vi "Escolher sinal.vi"(6 "Offset":dbl, 7 "Fase da onda":dbl, 9 "Numeric":dbl, 10 "Tipo de onda":T1, 11 "Amplitude":dbl) -> (3 "Sawtooth":dynamicdata(waveform))   [LabVIEW 2014]
uses:
  Tipos de onda.ctl
  <vilib>/measure/NI_MAPro.lvlib
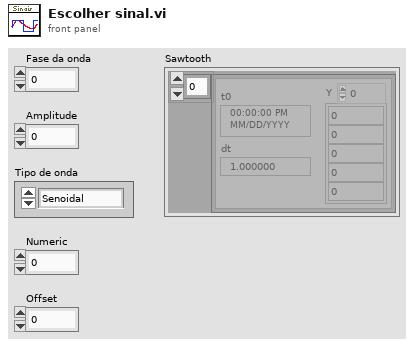
[diagram p1: front panel]
types:
  T1 = typedef "Tipos de onda.ctl" = enum16{"Senoidal", "Quadrada", "Triangular", "Trapezoidal", "Dente de Serra"}
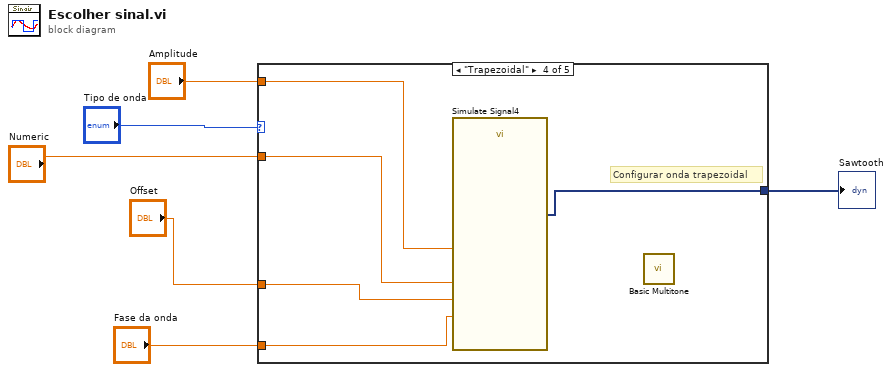
[diagram p0: block diagram]
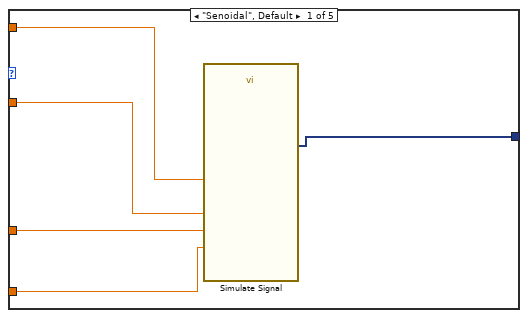
[diagram p2: hidden frame]
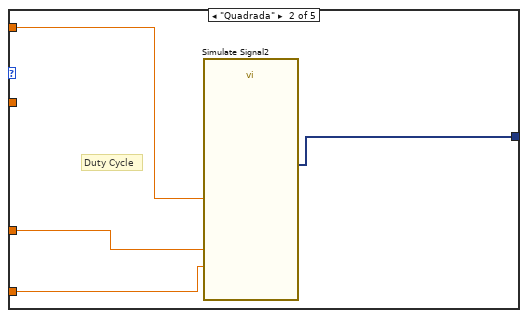
[diagram p3: hidden frame]
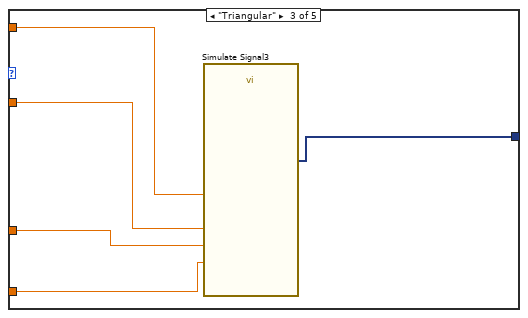
[diagram p4: hidden frame]
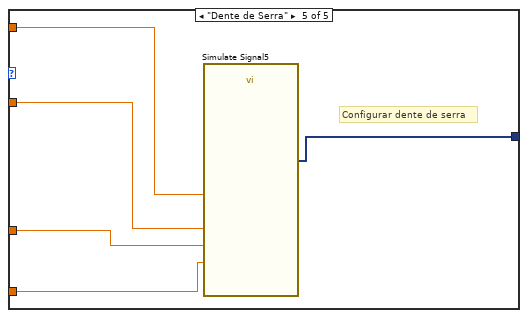
[diagram p5: hidden frame]
diagram:
  n1 = case shown="\"Trapezoidal\"" "Tipo de onda" {
    tunnel: "Amplitude" -> [w11 w15 w20 w25 w30]
    tunnel: "Numeric" -> [w10 _ w19 w24 w29]
    tunnel: "Fase da onda" -> [w9 w14 w18 w23 w28]
    tunnel: "Offset" -> [w8 w13 w17 w22 w27]
    tunnel: [w7 w12 w16 w21 w26] -> w6
    frame "Senoidal", Default {
      n2 = call "Simulate Signal"("Offset"=w8, "Frequency"=w10, "Amplitude"=w11, "Phase"=w9) -> ("Sine"=w7:dynamicdata)  [unwired: 10 in, 1 out]
    }
    frame "Quadrada" {
      # "Duty Cycle"
      n3 = call "Simulate Signal2"("Offset"=w13, "Amplitude"=w15, "Phase"=w14) -> ("Square"=w12:dynamicdata)  [unwired: 11 in, 1 out]
    }
    frame "Triangular" {
      n4 = call "Simulate Signal3"("Offset"=w17, "Frequency"=w19, "Amplitude"=w20, "Phase"=w18) -> ("Triangle"=w16:dynamicdata)  [unwired: 10 in, 1 out]
    }
    frame "Trapezoidal" {
      # "Configurar onda trapezoidal"
      n5 = call "Simulate Signal4"("Offset"=w22, "Frequency"=w24, "Amplitude"=w25, "Phase"=w23) -> ("Sine"=w21:dynamicdata)  [unwired: 10 in, 1 out]
      n6 = call <vilib>:"Basic Multitone.vi"() -> ()  [unwired: 12 in, 4 out]
    }
    frame "Dente de Serra" {
      # "Configurar dente de serra"
      n7 = call "Simulate Signal5"("Offset"=w27, "Frequency"=w29, "Amplitude"=w30, "Phase"=w28) -> ("Sawtooth"=w26:dynamicdata)  [unwired: 10 in, 1 out]
    }
  }
  "Sawtooth" <- w6
